vi "Pi-D (SubVI).vi"(0 "Desired Position":dbl, 1 "I Windup Limit":dbl=0.1, 5 "Actual Position":dbl, 7 "I Output Limit":dbl=0.1, 9 "Prop Gain":dbl, 11 "Int Gain":dbl, 12 "Deriv Gain":dbl) -> (4 "Output":dbl)   [LabVIEW 2015]
panel:
  out "Derivative":dbl
  out "Integral":dbl
  out "Proportional":dbl
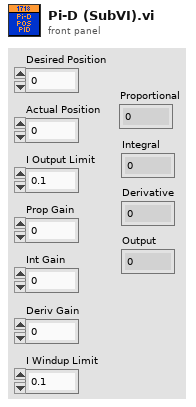
[diagram p1: front panel]
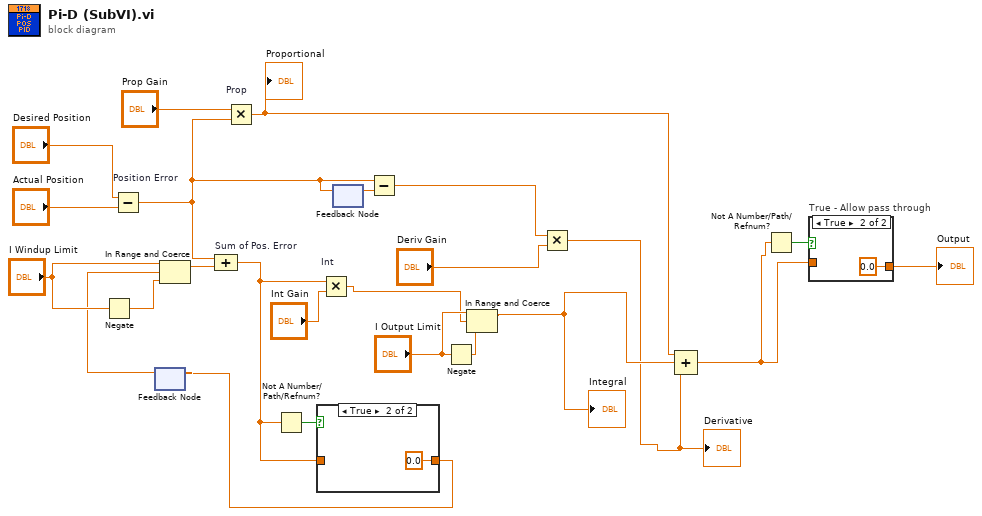
[diagram p0: block diagram]
diagram:
  n1 = Negate(x="I Windup Limit") -> (-x=w12:dbl)
  n2 = Subtract "Position Error"(x="Desired Position", y="Actual Position") -> (x-y=w15:dbl)
  n3 = feedback #1() -> (w10:dbl)  [unwired: 1 in]
  n4 = In Range and Coerce(upper limit="I Windup Limit", x=w10, lower limit=w12) -> (coerced(x)=w9:dbl)  [unwired: 1 out]
  n5 = Compound Arithmetic op=ADD "Sum of Pos. Error"(w15, w9) -> (w2:dbl)
  n6 = Multiply "Prop"(x="Prop Gain", y=w15) -> (x*y=w16:dbl)
  "Proportional" <- w16
  n7 = Not A Number/Path/Refnum?(number/path/refnum=w2) -> (NaN/Path/Refnum?=w3:bool)
  n8 = case shown="True" w3 {
    tunnel: w2 -> [w25 _]
    tunnel: [w25 0.0] -> w1
    frame False {
    }
    frame True {
    }
  }
  n9 = feedback-in #1(w1) -> ()
  n10 = Multiply "Int"(x=w2, y="Int Gain") -> (x*y=w8:dbl)
  n11 = feedback-in #2(w15) -> ()
  n12 = feedback #2() -> (w14:dbl)  [unwired: 1 in]
  n13 = Subtract(x=w15, y=w14) -> (x-y=w22:dbl)
  n14 = Negate(x="I Output Limit") -> (-x=w20:dbl)
  n15 = In Range and Coerce(upper limit="I Output Limit", x=w8, lower limit=w20) -> (coerced(x)=w13:dbl)  [unwired: 1 out]
  "Integral" <- w13
  n16 = Multiply(x=w22, y="Deriv Gain") -> (x*y=w7:dbl)
  "Derivative" <- w7
  n17 = Compound Arithmetic op=ADD(w16, w13, w7) -> (w4:dbl)
  n18 = Not A Number/Path/Refnum?(number/path/refnum=w4) -> (NaN/Path/Refnum?=w5:bool)
  n19 = case "True - Allow pass through" shown="True" w5 {
    tunnel: w4 -> [w27 _]
    tunnel: [w27 0.0] -> w6
    frame False {
    }
    frame True {
    }
  }
  "Output" <- w6
